vi "beta-4.0.0.vi"() -> ()   [LabVIEW 2016]
uses:
  output configuration.ctl
  <vilib>/FPGAPlugInAG/cRIO-9063/niLvFpga_Open_cRIO-9063.vi
  <vilib>/rvi/interface/common/dynamic/niFpgaDynamicAddResources.vi
  <vilib>/Utility/error.llb/Error Cluster From Error Code.vi
  <vilib>/rvi/errors/niLvFpgaAdjustHostInterfaceError.vi
  <vilib>/FPGAPlugInAG/Dynamic/niLvFpga_Close_Dynamic.vi
  <vilib>/rvi/interface/nirviOpenFPGA/nirviOpenFPGA.xnode
  FPGA Bitfiles/multi-functionpr_FPGATarget_multi-function-f_bsn-gyeHrfY.lvbitx
  multi-function-fpga-final.vi
  <vilib>/rvi/interface/nirviReadWriteControl/nirviReadWriteControl.xnode
  <vilib>/rvi/interface/nirviCloseFPGA/nirviCloseFPGA.xnode
  NiFpgaLv.dll
  <vilib>/rvi/interface/Simulation/niFpgaSimulationCallBeginRW.vi
panel:
  out "Change Indicator":bool[](array[boolean])
  in  "Output Configuration":T1[](array[typedef]) {"boolean high" format="%#_17g"; "boolean low" format="%#_17g"; "scan step" format="%#_17g"; "scan begin" format="%#_17g"; "scan end" format="%#_17g"}
  in  "Configure":bool
  in  "Load":bool
  out "State":enum16{"Loading", "Running"}(ring)
  # "channels from left to right corresponds to output0 to output15 of the box\n\nthere are  four functions:\nswitch: the main digital input will be treated as a switch, on - output boolean high; off - output boolean low\nand gate: main input and sub input will go through an and gate, then do as a switch\nor gate: main input and sub input will go through an or gate, then do as a switch\niteration: the output will iterate from scan begin by scan step when receive a main input pulse. When the voltage exceeds the scan end, the voltage will go back to the scan begin and start a new iteration. \n\nWarnning: the output voltage range is from -10V to +10V.\nWarnning: if you set a negtive step voltage, make sure begin voltage larger than end voltage, vice versa."
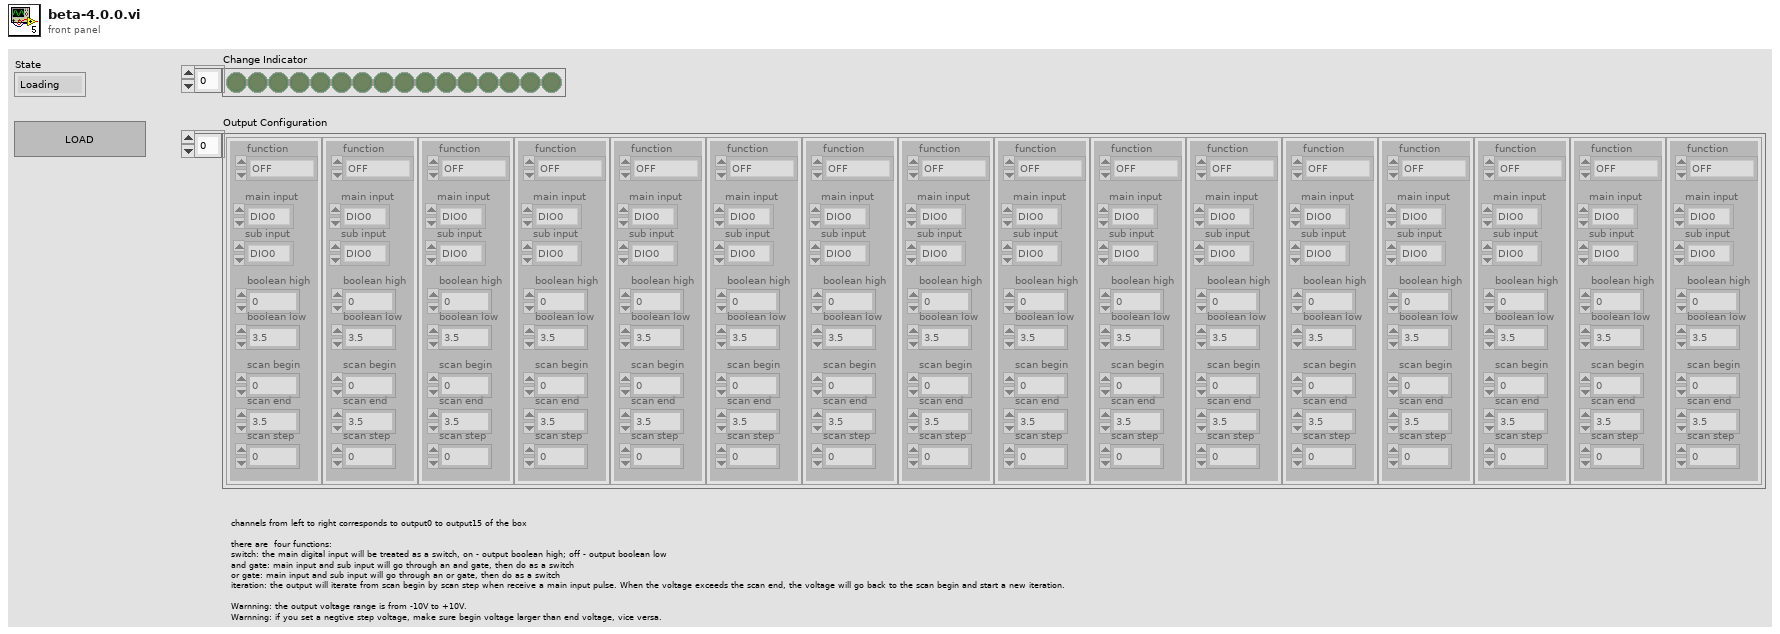
[diagram p1: front panel]
types:
  T1 = typedef "output configuration.ctl" = cluster{"function":enum16{"OFF", "SWITCH", "AND GATE", "OR GATE", "ITERATION"}, "scan end":sgl, "scan begin":sgl, "scan step":sgl, "main input":enum16{"DIO0", "DIO1", "DIO2", "DIO3", "DIO4", "DIO5", "DIO6", "DIO7", "DIO8", "DIO9", "DIO10", "DIO11", "DIO12", "DIO13", "DIO14", "DIO15", "DIO16", "DIO17", "DIO18", "DIO19", "DIO20", "DIO21", "DIO22", "DIO23", "DIO24", "DIO25", "DIO26", "DIO27", "DIO28", "DIO29", "DIO30", "DIO31"}, "sub input":enum16{"DIO0", "DIO1", "DIO2", "DIO3", "DIO4", "DIO5", "DIO6", "DIO7", "DIO8", "DIO9", "DIO10", "DIO11", "DIO12", "DIO13", "DIO14", "DIO15", "DIO16", "DIO17", "DIO18", "DIO19", "DIO20", "DIO21", "DIO22", "DIO23", "DIO24", "DIO25", "DIO26", "DIO27", "DIO28", "DIO29", "DIO30", "DIO31"}, "boolean low":sgl, "boolean high":sgl}
  T2 = cluster{"function":bool, "scan end":bool, "scan begin":bool, "scan step":bool, "main input":bool, "sub input":bool, "boolean low":bool, "boolean high":bool}[]
  T3 = cluster{"function":enum16{"OFF", "SWITCH", "AND GATE", "OR GATE", "ITERATION"}, "scan end":sgl, "scan begin":sgl, "scan step":sgl, "main input":enum16{"DIO0", "DIO1", "DIO2", "DIO3", "DIO4", "DIO5", "DIO6", "DIO7", "DIO8", "DIO9", "DIO10", "DIO11", "DIO12", "DIO13", "DIO14", "DIO15", "DIO16", "DIO17", "DIO18", "DIO19", "DIO20", "DIO21", "DIO22", "DIO23", "DIO24", "DIO25", "DIO26", "DIO27", "DIO28", "DIO29", "DIO30", "DIO31"}, "sub input":enum16{"DIO0", "DIO1", "DIO2", "DIO3", "DIO4", "DIO5", "DIO6", "DIO7", "DIO8", "DIO9", "DIO10", "DIO11", "DIO12", "DIO13", "DIO14", "DIO15", "DIO16", "DIO17", "DIO18", "DIO19", "DIO20", "DIO21", "DIO22", "DIO23", "DIO24", "DIO25", "DIO26", "DIO27", "DIO28", "DIO29", "DIO30", "DIO31"}, "boolean low":sgl, "boolean high":sgl, bool}[]
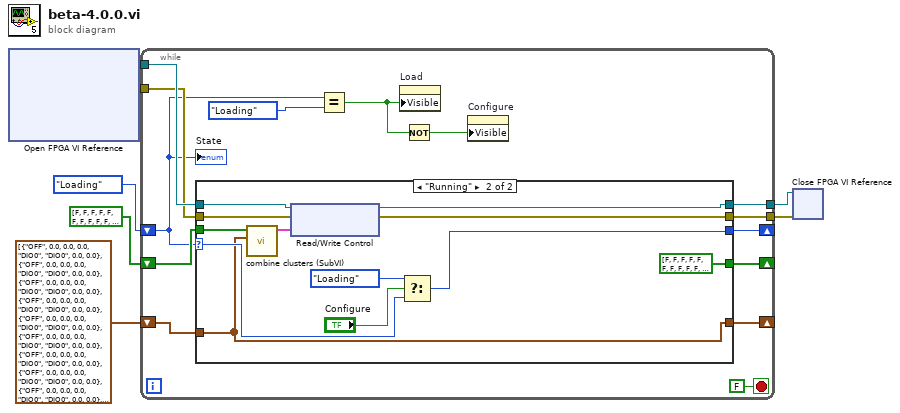
[diagram p0: block diagram]
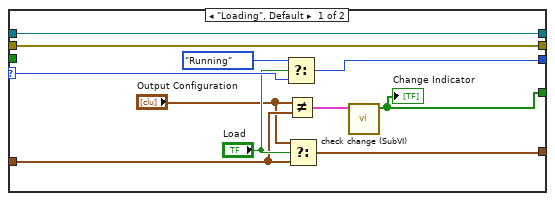
[diagram p2: hidden frame]
diagram:
  n1 = xnode "Open FPGA VI Reference"() -> ("FPGA VI Reference Out"=w3:refnum<k20>, "error out"=w2:errorcluster)  [unwired: 2 in]
  n2 = while {
    shift-right: [w19] -> _
    shift-left: T1[] [{"function"=enum."OFF", "scan end"=0.0, "scan begin"=0.0, "scan step"=0.0, "main input"=enum."DIO0", "sub input"=enum."DIO0", "boolean low"=0.0, "boolean high"=0.0}, {"function"=enum."OFF", "scan end"=0.0, "scan begin"=0.0, "scan step"=0.0, "main input"=enum."DIO0", "sub input"=enum."DIO0", "boolean low"=0.0, "boolean high"=0.0}, {"function"=enum."OFF", "scan end"=0.0, "scan begin"=0.0, "scan step"=0.0, "main input"=enum."DIO0", "sub input"=enum."DIO0", "boolean low"=0.0, "boolean high"=0.0}, {"function"=enum."OFF", "scan end"=0.0, "scan begin"=0.0, "scan step"=0.0, "main input"=enum."DIO0", "sub input"=enum."DIO0", "boolean low"=0.0, "boolean high"=0.0}, {"function"=enum."OFF", "scan end"=0.0, "scan begin"=0.0, "scan step"=0.0, "main input"=enum."DIO0", "sub input"=enum."DIO0", "boolean low"=0.0, "boolean high"=0.0}, {"function"=enum."OFF", "scan end"=0.0, "scan begin"=0.0, "scan step"=0.0, "main input"=enum."DIO0", "sub input"=enum."DIO0", "boolean low"=0.0, "boolean high"=0.0}, {"function"=enum."OFF", "scan end"=0.0, "scan begin"=0.0, "scan step"=0.0, "main input"=enum."DIO0", "sub input"=enum."DIO0", "boolean low"=0.0, "boolean high"=0.0}, {"function"=enum."OFF", "scan end"=0.0, "scan begin"=0.0, "scan step"=0.0, "main input"=enum."DIO0", "sub input"=enum."DIO0", "boolean low"=0.0, "boolean high"=0.0}, {"function"=enum."OFF", "scan end"=0.0, "scan begin"=0.0, "scan step"=0.0, "main input"=enum."DIO0", "sub input"=enum."DIO0", "boolean low"=0.0, "boolean high"=0.0}, {"function"=enum."OFF", "scan end"=0.0, "scan begin"=0.0, "scan step"=0.0, "main input"=enum."DIO0", "sub input"=enum."DIO0", "boolean low"=0.0, "boolean high"=0.0}, {"function"=enum."OFF", "scan end"=0.0, "scan begin"=0.0, "scan step"=0.0, "main input"=enum."DIO0", "sub input"=enum."DIO0", "boolean low"=0.0, "boolean high"=0.0}, {"function"=enum."OFF", "scan end"=0.0, "scan begin"=0.0, "scan step"=0.0, "main input"=enum."DIO0", "sub input"=enum."DIO0", "boolean low"=0.0, "boolean high"=0.0}, {"function"=enum."OFF", "scan end"=0.0, "scan begin"=0.0, "scan step"=0.0, "main input"=enum."DIO0", "sub input"=enum."DIO0", "boolean low"=0.0, "boolean high"=0.0}, {"function"=enum."OFF", "scan end"=0.0, "scan begin"=0.0, "scan step"=0.0, "main input"=enum."DIO0", "sub input"=enum."DIO0", "boolean low"=0.0, "boolean high"=0.0}, {"function"=enum."OFF", "scan end"=0.0, "scan begin"=0.0, "scan step"=0.0, "main input"=enum."DIO0", "sub input"=enum."DIO0", "boolean low"=0.0, "boolean high"=0.0}, {"function"=enum."OFF", "scan end"=0.0, "scan begin"=0.0, "scan step"=0.0, "main input"=enum."DIO0", "sub input"=enum."DIO0", "boolean low"=0.0, "boolean high"=0.0}] ("Output Configuration") -> [w18]
    shift-right: [w20] -> _
    shift-left: enum16{"Loading", "Running"}."Loading" ("State") -> [w11]
    shift-right: [w12] -> _
    shift-left: bool[] [FALSE, FALSE, FALSE, FALSE, FALSE, FALSE, FALSE, FALSE, FALSE, FALSE, FALSE, FALSE, FALSE, FALSE, FALSE, FALSE] -> [w13]
    tunnel: w3 -> [w17]
    tunnel: w2 -> [w16]
    tunnel: [w15] -> w6
    tunnel: [w14] -> w5
    stop <- FALSE stop-if-true
    n3 = case shown="\"Running\"" w11 {
      selector: w11 -> [w32 w41]
      tunnel: [w31 w43] -> w20
      tunnel: [w27 w35] -> w19
      tunnel: w18 -> [w28 w35]
      tunnel: [w22 bool[] [FALSE, FALSE, FALSE, FALSE, FALSE, FALSE, FALSE, FALSE, FALSE, FALSE, FALSE, FALSE, FALSE, FALSE, FALSE, FALSE]] -> w12
      tunnel: w17 -> [w26 w40]
      tunnel: w16 -> [w25 w39]
      tunnel: [w26 w38] -> w15
      tunnel: [w25 w37] -> w14
      tunnel: w13 -> [_ w34]
      frame "Loading", Default {
        n4 = Select(t=enum16{"Loading", "Running"}."Running", s="Load", f=w32) -> (s? t:f=w31:enum16{"Loading", "Running"})
        n5 = Not Equal?(x="Output Configuration", y=w28) -> (x != y?=w23:T2)
        n6 = Select(t="Output Configuration", s="Load", f=w28) -> (s? t:f=w27:T1[])
        n7 = call "check change (SubVI).vi"("Array in"=w23) -> ("Array out"=w22:bool[])  [unwired: 10 in]
        "Change Indicator" <- w22
      }
      frame "Running" {
        n8 = call "combine clusters (SubVI).vi"("Output Configuration"=w35, "Array in"=w34) -> ("Array out"=w33:T3)  [unwired: 9 in]
        n9 = xnode "Read/Write Control"("FPGA VI Reference In"=w40, "error in"=w39, "fpga controls"=w33) -> ("FPGA VI Reference Out"=w38:refnum<k20>, "error out"=w37:errorcluster)
        n10 = Select(t=enum16{"Loading", "Running"}."Loading", s="Configure", f=w41) -> (s? t:f=w43:enum16{"Loading", "Running"})
      }
    }
    n11 = Equal?(x=w11, y=enum16{"Loading", "Running"}."Loading") -> (x = y?=w8:bool)
    n12 = property on="Load" class="Bool"("Visible"=w8) -> ()  [unwired: 2 in, 2 out]
    n13 = Not(x=w8) -> (.not. x?=w9:bool)
    n14 = property on="Configure" class="Bool"("Visible"=w9) -> ()  [unwired: 2 in, 2 out]
    "State" <- w11
  }
  n15 = xnode "Close FPGA VI Reference"("FPGA VI Reference In"=w6, "error in"=w5) -> ()  [unwired: 1 out]
